vi "WLAN - TV - OPPO - CreateSingleTestVector.vi"(7 "TV_IQComposite_11AC":T7={"Standard"=4, "OFDM Advanced Controls"={"OFDM Auto Compute Acquisition Length Enabled"=0, "OFDM Maximum Symbols Used"=0, "OFDM Time Tracking Enabled"=0, "OFDM Channel Tracking Enabled"=0, "OFDM Amplitude Tracking Enabled"=1, "OFDM CFO Estimation Method"=0, "OFDM Phase Tracking Method"=0, "OFDM Header Detection Enabled"=0, "OFDM MAC FCS Check Enabled"=0, "#Avg"=10, "#Iterations"=10}, "Measurement Enabled"=TRUE, "#Packets"=0, "Center Frequency(Hz)"=0.0, "Guard Interval (s)"=0.0, "FEC Coding Type"=0, "Generation Parameters"={"Channel BW(Hz)"=20000000.0, "MCS Index"=0, "OFDM Payload Length (bytes)"=4024, "Idle Interval(S)"=0.0, "N_SS"=0}, "Power Level(dBm)"=0.0} {"Generation Parameters"."Channel BW(Hz)" items=["5M"=5000000.0, "10M"=10000000.0, "20M"=20000000.0, "40M"=40000000.0, "80M"=80000000.0, "160M"=160000000.0]; "FEC Coding Type" items=["BCC", "LDPC"]; "Center Frequency(Hz)" format="%#_6p"; "OFDM Advanced Controls"."OFDM Phase Tracking Method" items=["Standard", "Instantaneous", "None", "Standard with Cubic Spline Fit"]; "OFDM Advanced Controls"."OFDM CFO Estimation Method" items=["Preamble Only", "Preamble and Data"]; "OFDM Advanced Controls"."OFDM Channel Tracking Enabled" items=["False", "True"]; "OFDM Advanced Controls"."OFDM Amplitude Tracking Enabled" items=["False", "True"]; "OFDM Advanced Controls"."OFDM Time Tracking Enabled" items=["True"=1, "False"=0]; "OFDM Advanced Controls"."OFDM Auto Compute Acquisition Length Enabled" items=["False", "True"]; "OFDM Advanced Controls"."OFDM MAC FCS Check Enabled" items=["False", "True"]; "OFDM Advanced Controls"."OFDM Header Detection Enabled" items=["False", "True"]; "Standard" items=["80211A/G/J/P OFDM", "80211B/G DSSS", "80211G DSSSOFDM", "80211N MIMOOFDM", "80211AC MIMOOFDM"]}, 8 "TV_IQComposite_11N":T6={"Standard"=3, "OFDM Advanced Controls"={"OFDM Auto Compute Acquisition Length Enabled"=0, "OFDM Maximum Symbols Used"=0, "OFDM Time Tracking Enabled"=0, "OFDM Channel Tracking Enabled"=0, "OFDM Amplitude Tracking Enabled"=1, "OFDM CFO Estimation Method"=0, "OFDM Phase Tracking Method"=0, "OFDM Header Detection Enabled"=0, "OFDM MAC FCS Check Enabled"=0, "#Avg"=10, "#Iterations"=10}, "Measurement Enabled"=FALSE, "#Packets"=0, "Guard Interval (s)"=0.0, "FEC Coding Type"=0, "80211n PLCP Frame Format"=0, "Generation Parameters"={"Channel Bandwidth(Hz)"=20000000.0, "MCS Index"=0, "OFDM Payload Length (bytes)"=4024, "Idle Interval(S)"=0.0}, "Power Level(dBm)"=0.0, "Center Frequency(Hz)"=0.0} {"Center Frequency(Hz)" format="%#_6p"; "Generation Parameters"."Channel Bandwidth(Hz)" items=["5M"=5000000.0, "10M"=10000000.0, "20M"=20000000.0, "40M"=40000000.0, "80M"=80000000.0, "160M"=160000000.0]; "80211n PLCP Frame Format" items=["Mixed Format", "Greenfield Format"]; "FEC Coding Type" items=["BCC", "LDPC"]; "OFDM Advanced Controls"."OFDM Phase Tracking Method" items=["Standard", "Instantaneous", "None", "Standard with Cubic Spline Fit"]; "OFDM Advanced Controls"."OFDM CFO Estimation Method" items=["Preamble Only", "Preamble and Data"]; "OFDM Advanced Controls"."OFDM Channel Tracking Enabled" items=["False", "True"]; "OFDM Advanced Controls"."OFDM Amplitude Tracking Enabled" items=["False", "True"]; "OFDM Advanced Controls"."OFDM Time Tracking Enabled" items=["True"=1, "False"=0]; "OFDM Advanced Controls"."OFDM Auto Compute Acquisition Length Enabled" items=["False", "True"]; "OFDM Advanced Controls"."OFDM MAC FCS Check Enabled" items=["False", "True"]; "OFDM Advanced Controls"."OFDM Header Detection Enabled" items=["False", "True"]; "Standard" items=["80211A/G/J/P OFDM", "80211B/G DSSS", "80211G DSSSOFDM", "80211N MIMOOFDM", "80211AC MIMOOFDM"]}, 9 "TV_IQComposite_11B":T4={"Standard"=0, "DSSS Demod Parameters"={"DSSS Auto Compute Acquisition Length Enabled"=0, "DSSS Equalization Enabled"=0, "DSSS Header Detection Enabled"=0, "DSSS MAC FCS Check Enabled"=0, "DSSS Measurement Start Location"=0, "DSSS Phase Tracking Method"=0, "DSSS Maximum Chips Used"=0, "DSSS Reference Pulse Shaping Filter"=0, "DSSS Reference Pulse Shaping Filter Coefficient"=0.0, "# Avg"=1024, "# Iterations"=1024, "DSSS Power Ramp Enabled"=0}, "Measurement Enabled ? "=FALSE, "Power Level(dBm)"=0.0, "Center Frequency(Hz)"=0.0, "DSSS Generate Parameters"={"DSSS Data Rate (Mbps)"=0, "DSSS Payload Length (bytes)"=1024, "Idle Interval(S)"=0.0}} {"DSSS Generate Parameters"."DSSS Data Rate (Mbps)" items=["1", "2", "5.5 CCK", "5.5 PBCC", "11 CCK", "11 PBCC", "22", "33"]; "Center Frequency(Hz)" format="%#_6p"; "DSSS Demod Parameters"."DSSS Power Ramp Enabled" items=["False", "True"]; "DSSS Demod Parameters"."DSSS Auto Compute Acquisition Length Enabled" items=["False", "True"]; "DSSS Demod Parameters"."DSSS Phase Tracking Method" items=["Standard", "Instantaneous"]; "DSSS Demod Parameters"."DSSS Equalization Enabled" items=["False", "True"]; "DSSS Demod Parameters"."DSSS Reference Pulse Shaping Filter" items=["Rectangular", "Raised Cosine", "Root Raised Cosine", "Gaussian"]; "DSSS Demod Parameters"."DSSS MAC FCS Check Enabled" items=["False", "True"]; "DSSS Demod Parameters"."DSSS Header Detection Enabled" items=["False", "True"]; "Standard" items=["80211A/G/J/P OFDM", "80211B/G DSSS", "80211G DSSSOFDM", "80211N MIMOOFDM", "80211AC MIMOOFDM"]}, 10 "Standard":T1(tab)=enum."80211GDSSSOFDM", 11 "IQComp_11AG OFDM":T2={"Standard"=0, "OFDM Advanced Controls"={"OFDM Auto Compute Acquisition Length Enabled"=0, "OFDM Maximum Symbols Used"=0, "OFDM Time Tracking Enabled"=0, "OFDM Channel Tracking Enabled"=0, "OFDM Amplitude Tracking Enabled"=1, "OFDM CFO Estimation Method"=0, "OFDM Phase Tracking Method"=0, "OFDM Header Detection Enabled"=0, "OFDM MAC FCS Check Enabled"=0, "#Avg"=0, "#Iterations"=10}, "Measurement  Enabled ?"=FALSE, "#Packets"=0, "Center Frequency(Hz)"=0.0, "Power Level(dBm)"=0.0, "Payload Control"={"OFDM Data Rate (Mbps)"=0, "OFDM Payload Length (bytes)"=0, "Idle Interval (s)"=0.0}} {"Payload Control"."OFDM Data Rate (Mbps)" items=["6", "9", "12", "18", "24", "36", "48", "54"]; "Center Frequency(Hz)" format="%#_6p"; "OFDM Advanced Controls"."OFDM Phase Tracking Method" items=["Standard", "Instantaneous", "None", "Standard with Cubic Spline Fit"]; "OFDM Advanced Controls"."OFDM CFO Estimation Method" items=["Preamble Only", "Preamble and Data"]; "OFDM Advanced Controls"."OFDM Channel Tracking Enabled" items=["False", "True"]; "OFDM Advanced Controls"."OFDM Amplitude Tracking Enabled" items=["False", "True"]; "OFDM Advanced Controls"."OFDM Time Tracking Enabled" items=["True"=1, "False"=0]; "OFDM Advanced Controls"."OFDM Auto Compute Acquisition Length Enabled" items=["False", "True"]; "OFDM Advanced Controls"."OFDM MAC FCS Check Enabled" items=["False", "True"]; "OFDM Advanced Controls"."OFDM Header Detection Enabled" items=["False", "True"]; "Standard" items=["80211A/G/J/P OFDM", "80211B/G DSSS", "80211G DSSSOFDM", "80211N MIMOOFDM", "80211AC MIMOOFDM"]}) -> (1 "WLAN Measurement Settings":T8={"OFDM Advanced Controls(11ag)"={"OFDM Auto Compute Acquisition Length Enabled"=0, "OFDM Maximum Symbols Used"=0, "OFDM Time Tracking Enabled"=0, "OFDM Channel Tracking Enabled"=0, "OFDM Amplitude Tracking Enabled"=1, "OFDM CFO Estimation Method"=0, "OFDM Phase Tracking Method"=0, "OFDM Header Detection Enabled"=0, "OFDM MAC FCS Check Enabled"=0, "#Avg"=10, "#Iterations"=10}, "DSSS Demod Parameters"={"DSSS Auto Compute Acquisition Length Enabled"=0, "DSSS Equalization Enabled"=0, "DSSS Header Detection Enabled"=0, "DSSS MAC FCS Check Enabled"=0, "DSSS Measurement Start Location"=0, "DSSS Phase Tracking Method"=0, "DSSS Maximum Chips Used"=0, "DSSS Reference Pulse Shaping Filter"=0, "DSSS Reference Pulse Shaping Filter Coefficient"=0.0, "# Avg"=1024, "# Iterations"=1024, "DSSS Power Ramp Enabled"=0}, "OFDM Advanced Controls (11n)"={"OFDM Auto Compute Acquisition Length Enabled"=0, "OFDM Maximum Symbols Used"=0, "OFDM Time Tracking Enabled"=0, "OFDM Channel Tracking Enabled"=0, "OFDM Amplitude Tracking Enabled"=1, "OFDM CFO Estimation Method"=0, "OFDM Phase Tracking Method"=0, "OFDM Header Detection Enabled"=0, "OFDM MAC FCS Check Enabled"=0, "#Avg"=10, "#Iterations"=10}, "OFDM Advanced Controls(11ac)"={"OFDM Auto Compute Acquisition Length Enabled"=0, "OFDM Maximum Symbols Used"=0, "OFDM Time Tracking Enabled"=1, "OFDM Channel Tracking Enabled"=0, "OFDM Amplitude Tracking Enabled"=0, "OFDM CFO Estimation Method"=0, "OFDM Phase Tracking Method"=0, "OFDM Header Detection Enabled"=0, "OFDM MAC FCS Check Enabled"=0, "#Avg"=10, "#Iterations"=10}} {"OFDM Advanced Controls(11ac)"."OFDM Phase Tracking Method" items=["Standard", "Instantaneous", "None", "Standard with Cubic Spline Fit"]; "OFDM Advanced Controls(11ac)"."OFDM CFO Estimation Method" items=["Preamble Only", "Preamble and Data"]; "OFDM Advanced Controls(11ac)"."OFDM Channel Tracking Enabled" items=["False", "True"]; "OFDM Advanced Controls(11ac)"."OFDM Amplitude Tracking Enabled" items=["False", "True"]; "OFDM Advanced Controls(11ac)"."OFDM Time Tracking Enabled" items=["True"=1, "False"=0]; "OFDM Advanced Controls(11ac)"."OFDM Auto Compute Acquisition Length Enabled" items=["False", "True"]; "OFDM Advanced Controls(11ac)"."OFDM MAC FCS Check Enabled" items=["False", "True"]; "OFDM Advanced Controls(11ac)"."OFDM Header Detection Enabled" items=["False", "True"]; "OFDM Advanced Controls (11n)"."OFDM Phase Tracking Method" items=["Standard", "Instantaneous", "None", "Standard with Cubic Spline Fit"]; "OFDM Advanced Controls (11n)"."OFDM CFO Estimation Method" items=["Preamble Only", "Preamble and Data"]; "OFDM Advanced Controls (11n)"."OFDM Channel Tracking Enabled" items=["False", "True"]; "OFDM Advanced Controls (11n)"."OFDM Amplitude Tracking Enabled" items=["False", "True"]; "OFDM Advanced Controls (11n)"."OFDM Time Tracking Enabled" items=["True"=1, "False"=0]; "OFDM Advanced Controls (11n)"."OFDM Auto Compute Acquisition Length Enabled" items=["False", "True"]; "OFDM Advanced Controls (11n)"."OFDM MAC FCS Check Enabled" items=["False", "True"]; "OFDM Advanced Controls (11n)"."OFDM Header Detection Enabled" items=["False", "True"]; "DSSS Demod Parameters"."DSSS Power Ramp Enabled" items=["False", "True"]; "DSSS Demod Parameters"."DSSS Auto Compute Acquisition Length Enabled" items=["False", "True"]; "DSSS Demod Parameters"."DSSS Phase Tracking Method" items=["Standard", "Instantaneous"]; "DSSS Demod Parameters"."DSSS Equalization Enabled" items=["False", "True"]; "DSSS Demod Parameters"."DSSS Reference Pulse Shaping Filter" items=["Rectangular", "Raised Cosine", "Root Raised Cosine", "Gaussian"]; "DSSS Demod Parameters"."DSSS MAC FCS Check Enabled" items=["False", "True"]; "DSSS Demod Parameters"."DSSS Header Detection Enabled" items=["False", "True"]; "OFDM Advanced Controls(11ag)"."OFDM Phase Tracking Method" items=["Standard", "Instantaneous", "None", "Standard with Cubic Spline Fit"]; "OFDM Advanced Controls(11ag)"."OFDM CFO Estimation Method" items=["Preamble Only", "Preamble and Data"]; "OFDM Advanced Controls(11ag)"."OFDM Channel Tracking Enabled" items=["False", "True"]; "OFDM Advanced Controls(11ag)"."OFDM Amplitude Tracking Enabled" items=["False", "True"]; "OFDM Advanced Controls(11ag)"."OFDM Time Tracking Enabled" items=["True"=1, "False"=0]; "OFDM Advanced Controls(11ag)"."OFDM Auto Compute Acquisition Length Enabled" items=["False", "True"]; "OFDM Advanced Controls(11ag)"."OFDM MAC FCS Check Enabled" items=["False", "True"]; "OFDM Advanced Controls(11ag)"."OFDM Header Detection Enabled" items=["False", "True"]}, 2 "Tv Element":T9 {"Standard" items=["80211A/G/J/P OFDM", "80211B/G DSSS", "80211G DSSSOFDM", "80211N MIMOOFDM", "80211AC MIMOOFDM"]; "OFDM Data Rate (Mbps)" items=["6", "9", "12", "18", "24", "36", "48", "54"]; "80211n PLCP Frame Format" items=["Mixed Format", "Greenfield Format"]; "FEC Coding Type" items=["BCC", "LDPC"]; "DSSS Data Rate (Mbps)" items=["1", "2", "5.5 CCK", "5.5 PBCC", "11 CCK", "11 PBCC", "22", "33"]})   [LabVIEW 2012]
uses:
  RW/Includes/WLAN - TV - RW - INC - TV_DataType_Cluster.ctl
  RW/Includes/WLAN - TV - RW - INC - Tx_Measurement_Cluster.ctl
  RW/Includes/WLAN - TV - RW - INC - TV_OFDM Demod.ctl
  RW/Includes/WLAN - TV - RW - INC - TV_DSSS Demod.ctl
  RW/Includes/WLAN - TV - OPPO - RW - INC - TV_IQComposite_11A.ctl
  RW/Includes/WLAN - TV - OPPO - RW - INC - TV_IQComposite_11AC.ctl
  RW/Includes/WLAN - TV - OPPO - RW - INC - TV_IQComposite_11B.ctl
  RW/Includes/WLAN - TV - OPPO - RW - INC - TV_IQComposite_11N.ctl
  RW/Includes/WLAN - TV - RW - INC - TV_Parameters.ctl
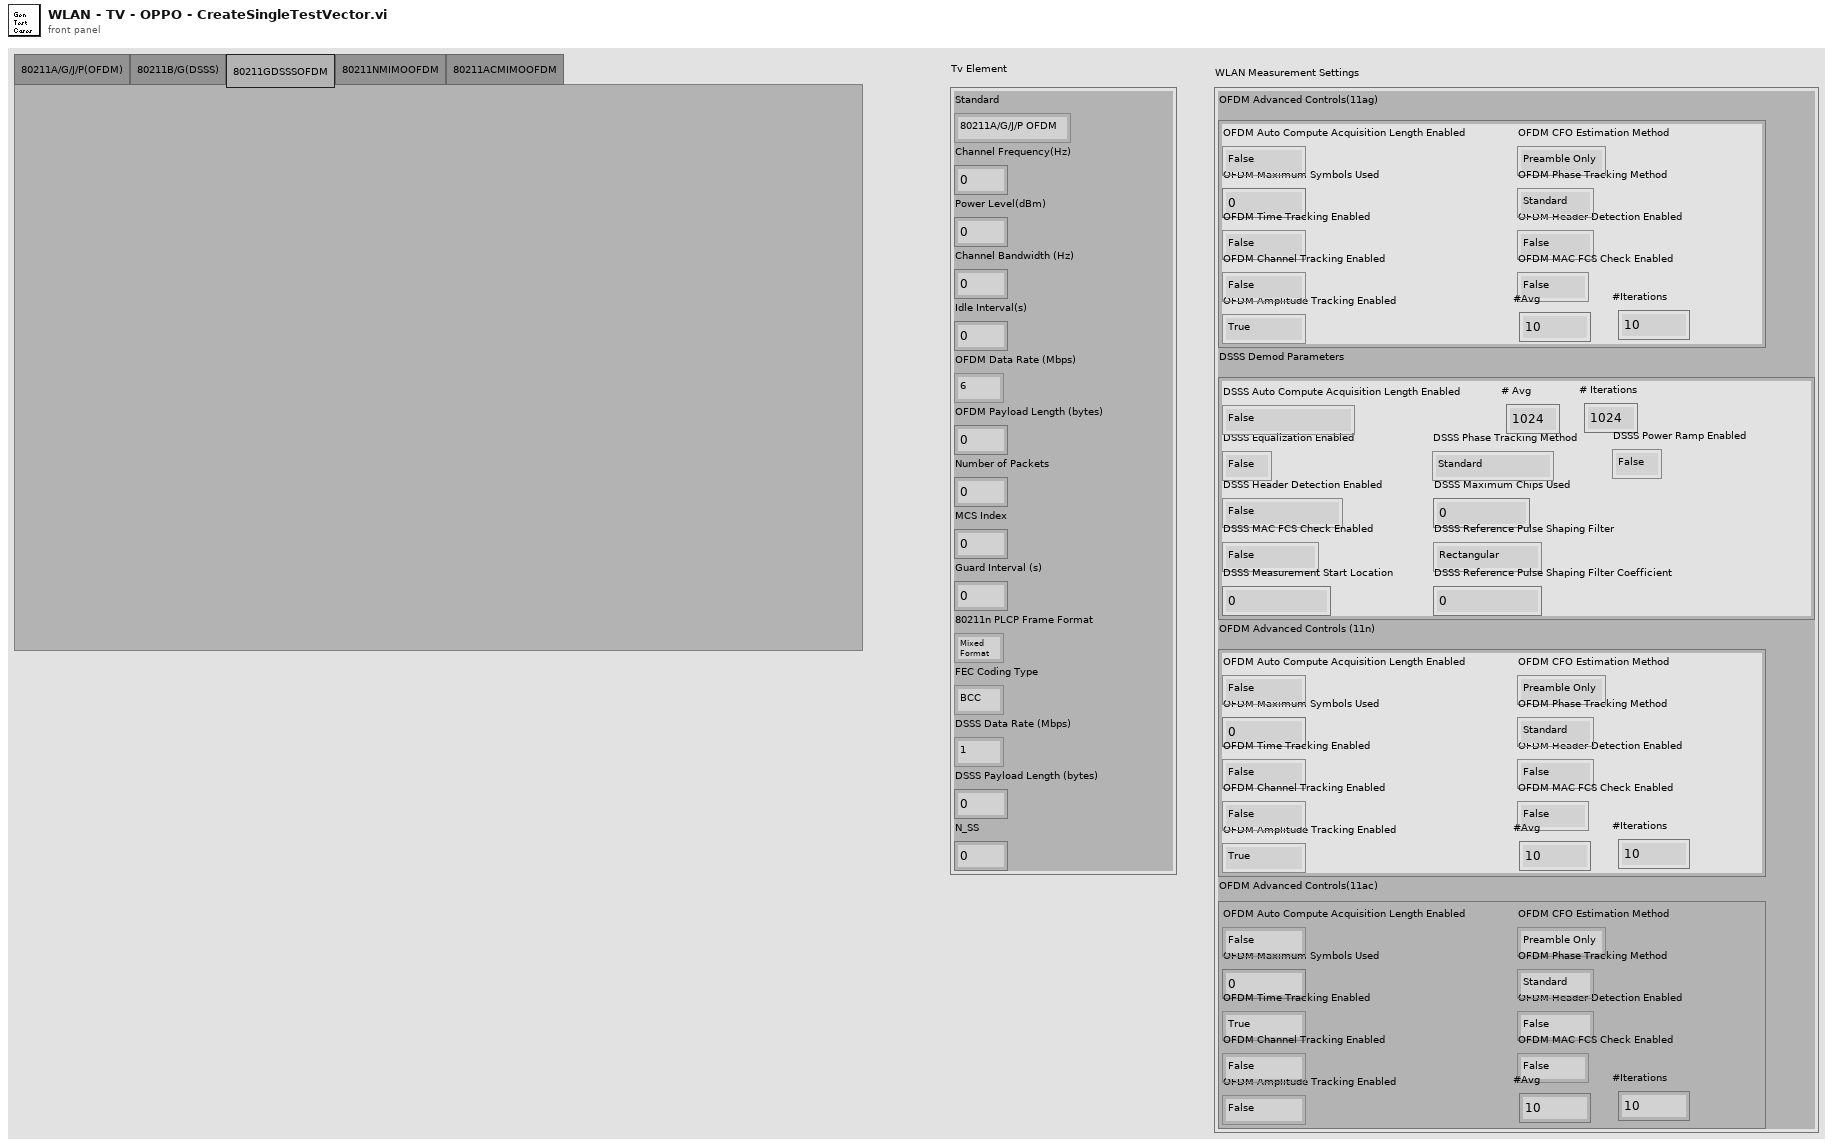
[diagram p1: front panel]
types:
  T1 = enum32{"80211A/G/J/P(OFDM)", "80211B/G(DSSS)", "80211GDSSSOFDM", "80211NMIMOOFDM", "80211ACMIMOOFDM"}
  T2 = typedef "WLAN - TV - OPPO - RW - INC - TV_IQComposite_11A.ctl" = cluster{"Standard":i32, "OFDM Advanced Controls":T3, "Measurement  Enabled ?":bool, "#Packets":i32, "Center Frequency(Hz)":dbl, "Power Level(dBm)":dbl, "Payload Control":cluster{"OFDM Data Rate (Mbps)":i32, "OFDM Payload Length (bytes)":i32, "Idle Interval (s)":dbl}}
  T3 = typedef "WLAN - TV - RW - INC - TV_OFDM Demod.ctl" = cluster{"OFDM Auto Compute Acquisition Length Enabled":i32, "OFDM Maximum Symbols Used":i32, "OFDM Time Tracking Enabled":i32, "OFDM Channel Tracking Enabled":i32, "OFDM Amplitude Tracking Enabled":i32, "OFDM CFO Estimation Method":i32, "OFDM Phase Tracking Method":i32, "OFDM Header Detection Enabled":i32, "OFDM MAC FCS Check Enabled":i32, "#Avg":i32, "#Iterations":i32}
  T4 = typedef "WLAN - TV - OPPO - RW - INC - TV_IQComposite_11B.ctl" = cluster{"Standard":i32, "DSSS Demod Parameters":T5, "Measurement Enabled ? ":bool, "Power Level(dBm)":dbl, "Center Frequency(Hz)":dbl, "DSSS Generate Parameters":cluster{"DSSS Data Rate (Mbps)":i32, "DSSS Payload Length (bytes)":i32, "Idle Interval(S)":dbl}}
  T5 = typedef "WLAN - TV - RW - INC - TV_DSSS Demod.ctl" = cluster{"DSSS Auto Compute Acquisition Length Enabled":i32, "DSSS Equalization Enabled":i32, "DSSS Header Detection Enabled":i32, "DSSS MAC FCS Check Enabled":i32, "DSSS Measurement Start Location":i32, "DSSS Phase Tracking Method":i32, "DSSS Maximum Chips Used":i32, "DSSS Reference Pulse Shaping Filter":i32, "DSSS Reference Pulse Shaping Filter Coefficient":dbl, "# Avg":i32, "# Iterations":i32, "DSSS Power Ramp Enabled":i32}
  T6 = typedef "WLAN - TV - OPPO - RW - INC - TV_IQComposite_11N.ctl" = cluster{"Standard":i32, "OFDM Advanced Controls":T3, "Measurement Enabled":bool, "#Packets":i32, "Guard Interval (s)":dbl, "FEC Coding Type":i32, "80211n PLCP Frame Format":i32, "Generation Parameters":cluster{"Channel Bandwidth(Hz)":dbl, "MCS Index":i32, "OFDM Payload Length (bytes)":i32, "Idle Interval(S)":dbl}, "Power Level(dBm)":dbl, "Center Frequency(Hz)":dbl}
  T7 = typedef "WLAN - TV - OPPO - RW - INC - TV_IQComposite_11AC.ctl" = cluster{"Standard":i32, "OFDM Advanced Controls":T3, "Measurement Enabled":bool, "#Packets":i32, "Center Frequency(Hz)":dbl, "Guard Interval (s)":dbl, "FEC Coding Type":i32, "Generation Parameters":cluster{"Channel BW(Hz)":dbl, "MCS Index":i32, "OFDM Payload Length (bytes)":i32, "Idle Interval(S)":dbl, "N_SS":i32}, "Power Level(dBm)":dbl}
  T8 = typedef "WLAN - TV - RW - INC - Tx_Measurement_Cluster.ctl" = cluster{"OFDM Advanced Controls(11ag)":T3, "DSSS Demod Parameters":T5, "OFDM Advanced Controls (11n)":T3, "OFDM Advanced Controls(11ac)":cluster{"OFDM Auto Compute Acquisition Length Enabled":i32, "OFDM Maximum Symbols Used":i32, "OFDM Time Tracking Enabled":i32, "OFDM Channel Tracking Enabled":i32, "OFDM Amplitude Tracking Enabled":i32, "OFDM CFO Estimation Method":i32, "OFDM Phase Tracking Method":i32, "OFDM Header Detection Enabled":i32, "OFDM MAC FCS Check Enabled":i32, "#Avg":i32, "#Iterations":i32}}
  T9 = typedef "WLAN - TV - RW - INC - TV_DataType_Cluster.ctl" = cluster{"Standard":i32, "Channel Frequency(Hz)":dbl, "Power Level(dBm)":dbl, "Channel Bandwidth (Hz)":dbl, "Idle Interval(s)":dbl, "OFDM Data Rate (Mbps)":i32, "OFDM Payload Length (bytes)":i32, "Number of Packets":i32, "MCS Index":i32, "Guard Interval (s)":dbl, "80211n PLCP Frame Format":i32, "FEC Coding Type":i32, "DSSS Data Rate (Mbps)":i32, "DSSS Payload Length (bytes)":i32, "N_SS":i32}
  T10 = typedef "WLAN - TV - RW - INC - TV_Parameters.ctl" = cluster{"Standard ":string, "Channel Frequency(Hz)":string, "Power Level(dBm)":string, "Channel Bandwidth (Hz)":string, "Idle Interval (s)":string, "OFDM Data Rate (Mbps)":string, "OFDM Payload Length (bytes)":string, "MCS Index":string, "Guard Interval (s)":string, "80211n PLCP Frame Format":string, "FEC Coding Type":string, "DSSS Data Rate (Mbps)":string, "DSSS Payload Length (bytes)":string, "#Packets":string, "N_SS":string}
  T11 = cluster{"IQComp_11AG OFDM":T2, "TV_IQComposite_11B":T4, "TV_IQComposite_11N":T6, "TV_IQComposite_11AC":T7}
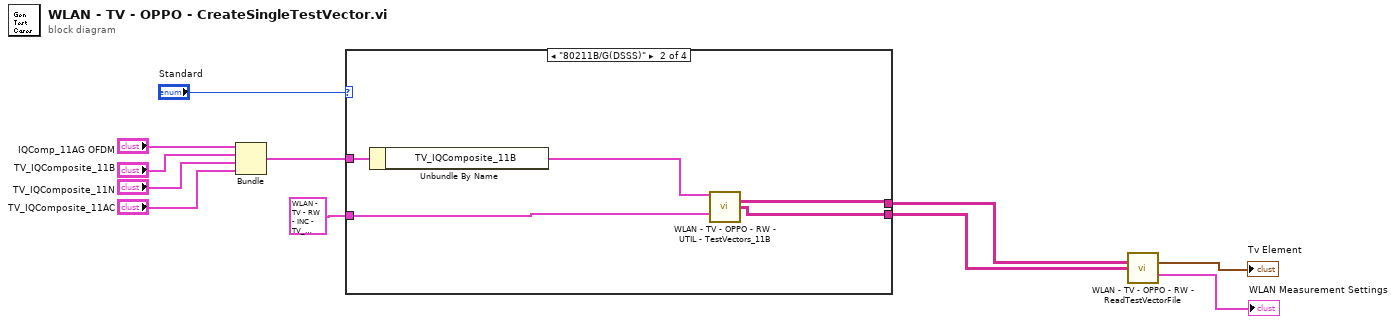
[diagram p0: block diagram]
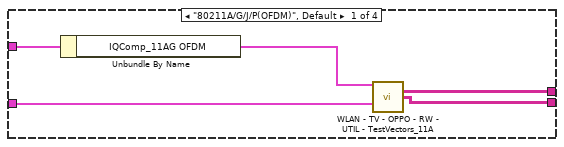
[diagram p2: hidden frame]
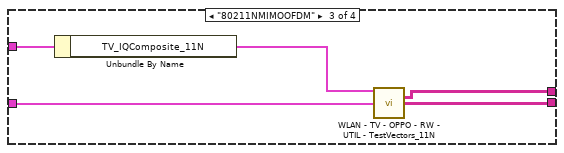
[diagram p3: hidden frame]
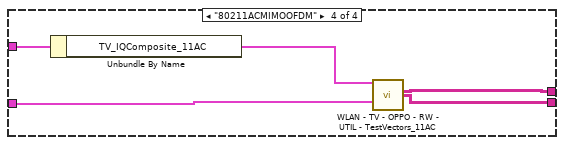
[diagram p4: hidden frame]
diagram:
  n1 = Bundle("IQComp_11AG OFDM"="IQComp_11AG OFDM", "TV_IQComposite_11B"="TV_IQComposite_11B", "TV_IQComposite_11N"="TV_IQComposite_11N", "TV_IQComposite_11AC"="TV_IQComposite_11AC") -> (w11:T11)  [unwired: 1 in]
  n2 = case shown="\"80211B/G(DSSS)\"" "Standard" {
    tunnel: w11 -> [w16 w21 w26 w31]
    tunnel: T10 {"Standard "="", "Channel Frequency(Hz)"="", "Power Level(dBm)"="", "Channel Bandwidth (Hz)"="", "Idle Interval (s)"="", "OFDM Data Rate (Mbps)"="", "OFDM Payload Length (bytes)"="", "MCS Index"="", "Guard Interval (s)"="", "80211n PLCP Frame Format"="", "FEC Coding Type"="", "DSSS Data Rate (Mbps)"="", "DSSS Payload Length (bytes)"="", "#Packets"="", "N_SS"=""} ("TV Paramaters") -> [w15 w20 w25 w30]
    tunnel: [w13 w18 w23 w27] -> w8
    tunnel: [w12 w17 w22 w28] -> w7
    frame "80211A/G/J/P(OFDM)", Default {
      n3 = Unbundle By Name(w16) -> ("IQComp_11AG OFDM"=w14:T2)
      n4 = call "WLAN - TV - OPPO - RW - UTIL - TestVectors_11A.vi"("IQComp_11AG OFDM"=w14, "TV Paramaters"=w15) -> ("TV"=w13:string[][], "Measure Config"=w12:string[][])  [unwired: 12 in]
    }
    frame "80211B/G(DSSS)" {
      n5 = Unbundle By Name(w21) -> ("TV_IQComposite_11B"=w19:T4)
      n6 = call "WLAN - TV - OPPO - RW - UTIL - TestVectors_11B.vi"("TV_IQComposite_11B"=w19, "TV Paramaters"=w20) -> ("TV"=w18:string[][], "Measure Config"=w17:string[][])  [unwired: 12 in]
    }
    frame "80211NMIMOOFDM" {
      n7 = Unbundle By Name(w26) -> ("TV_IQComposite_11N"=w24:T6)
      n8 = call "WLAN - TV - OPPO - RW - UTIL - TestVectors_11N.vi"("TV_IQComposite_11N"=w24, "TV Paramaters"=w25) -> ("TV"=w23:string[][], "Measure Config"=w22:string[][])  [unwired: 12 in]
    }
    frame "80211ACMIMOOFDM" {
      n9 = Unbundle By Name(w31) -> ("TV_IQComposite_11AC"=w29:T7)
      n10 = call "WLAN - TV - OPPO - RW - UTIL - TestVectors_11AC.vi"("TV_IQComposite_11AC"=w29, "TV Paramaters"=w30) -> ("TV"=w27:string[][], "Measure Config"=w28:string[][])  [unwired: 12 in]
    }
  }
  n11 = call "WLAN - TV - OPPO - RW - ReadTestVectorFile.vi"("TV"=w8, "Measure Config"=w7) -> ("Tv First Element"=→"Tv Element":T9, "WLAN Measurement Settings"=→"WLAN Measurement Settings":T8)  [unwired: 11 in, 1 out]
